vi "Call_Block_plug_ins.vi"(0 "Per Block Plug Ins":string[](array[string])) -> ()   [LabVIEW 2021]
uses:
  Globals/Dynamic_call_global.ph.vi
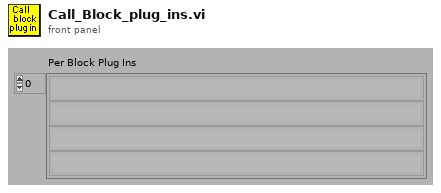
[diagram p1: front panel]
types:
  T1 = enum32{"Invalid", "Standard", "Closed", "Hidden", "Minimized", "Maximized"}
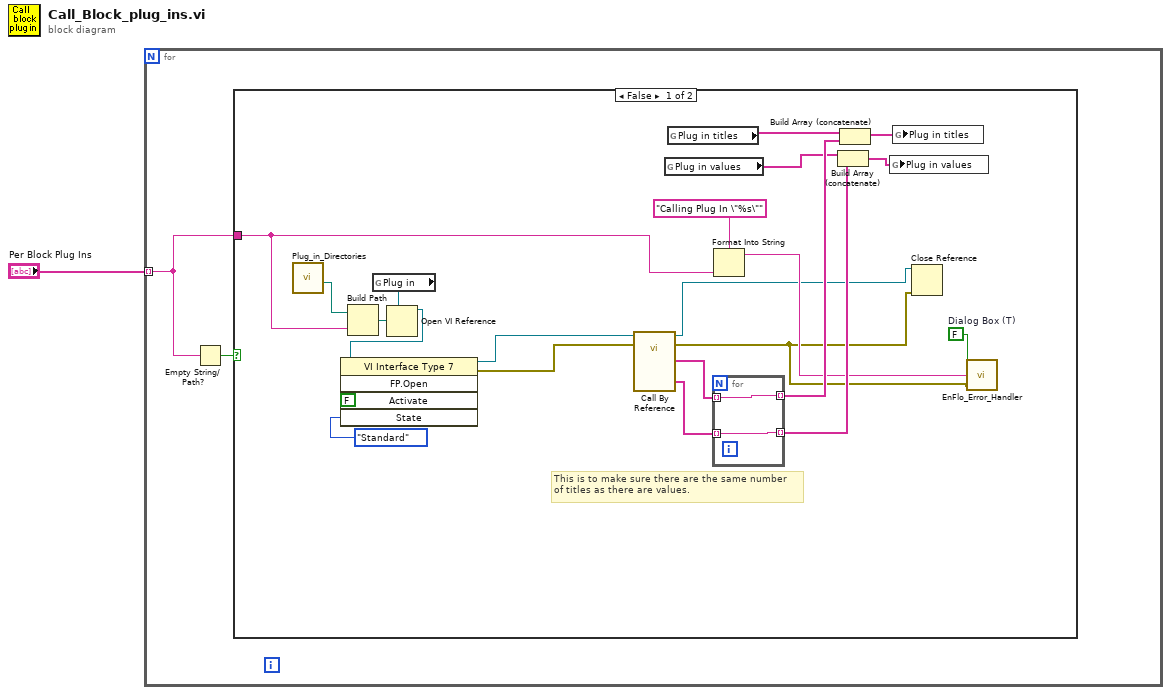
[diagram p0: block diagram]
diagram:
  n1 = for {
    tunnel: "Per Block Plug Ins" -> [w3] mode=indexing
    n2 = Empty String/Path?(string/path=w3) -> (empty?=w2:bool)
    n3 = case shown="False" w2 {
      tunnel: w3 -> [w4 _]
      frame False {
        w19 = FALSE  # Dialog Box (T)
        # "This is to make sure there are the same number\nof titles as there are values."
        n4 = call "Plug_in_Directories.vi"() -> ("Per Block"=w12:path)  [unwired: 2 in, 4 out]
        n5 = Build Path(base path=w12, name or relative path=w4) -> (appended path=w10:path)
        n6 = global read "Dynamic_call_global.ph.vi" "Plug in"() -> (w11:refnum<vi>)
        n7 = Open VI Reference(type specifier VI Refnum (for type only)=w11, vi path=w10) -> (vi reference=w9:refnum<vi>)  [unwired: 2 in, 3 out]
        n8 = invoke class="VI Interface Type 7" method="FP.Open"(reference=w9, "Activate"=FALSE ("Activate?"), "State"=T1."Standard") -> (reference out=w20:refnum<vi>, error out=w21:errorcluster)  [unwired: 2 in, 3 out]
        n9 = call-by-ref "?"(reference=w20, error in=w21) -> (reference out=w5:refnum<vi>, error out=w6:errorcluster, "Plug in titles"=w24:string[], "Plug in values"=w22:string[])  [unwired: 6 in]
        n10 = global read "Dynamic_call_global.ph.vi" "Plug in values"() -> (w18:string[])
        n11 = global read "Dynamic_call_global.ph.vi" "Plug in titles"() -> (w17:string[])
        n12 = for {
          tunnel: [w27] -> w25 mode=indexing
          tunnel: w24 -> [w27] mode=indexing
          tunnel: [w26] -> w23 mode=indexing
          tunnel: w22 -> [w26] mode=indexing
        }
        n13 = Format Into String(format string="Calling Plug In \"%s\"" ("Error Type"), w4) -> (resulting string=w13:string)  [unwired: 2 in, 1 out]
        n14 = Build Array (concatenate)(w18, w23) -> (w16:string[])
        n15 = Build Array (concatenate)(w17, w25) -> (w15:string[])
        n16 = global write "Dynamic_call_global.ph.vi" "Plug in values"(w16) -> ()
        n17 = global write "Dynamic_call_global.ph.vi" "Plug in titles"(w15) -> ()
        n18 = Close Reference(reference=w5, error in (no error)=w6) -> ()  [unwired: 1 out]
        n19 = call "EnFlo_Error_Handler.vi"("error in (no error)"=w6, "Error Type"=w13, "Dialog Box (F)"=w19) -> ()  [unwired: 3 out]
      }
      frame True {
      }
    }
  }
